vi "Open Log File Instance.vi"(8 "error in (no error)":errorcluster, 11 "Segmented Log in":refnum<class "Segmented Log.lvclass">) -> (0 "error out":errorcluster, 3 "Segmented Log out":refnum<class "Segmented Log.lvclass">)   [LabVIEW 2015, in "Waveform Data Logger Engine.lvlib" / "Segmented Log.lvclass"]
doc: "This VI opens a new log file instance based on the Log File Specification if the max number of instances has not yet been reached. This VI also notifies any listeners that a new file has been opened. If the max number of instances has already been met, this VI throws an error.\n\nBefore opening the file this VI updates the Instance and CrashFileInstance path tags. The Instance tag represents the one-based file index that the segmented log is about to open. The CrashFileInstance is a number that toggles between one and two. Using this tag allows users to create a crash log file session, which always records a running set of the most recent data to file, so that the last N samples are available in the case of a crash."
uses:
  Segmented Log.lvclass
  Shared/Classes/Log File Specifications/Log File Specification/Log File Specification.lvclass
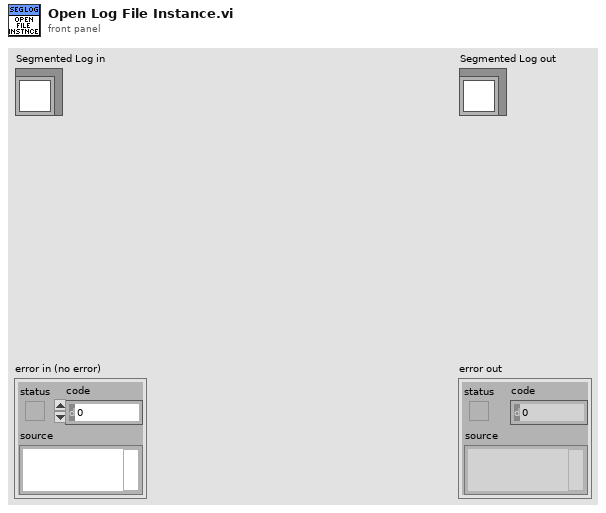
[diagram p1: front panel]
types:
  T1 = typedef "Waveform Data Logger Engine.lvlib/Segmented Log.lvclass/File Open Event Registration.ctl" = cluster{"Callback":refnum<vi>, "User Data":variant}
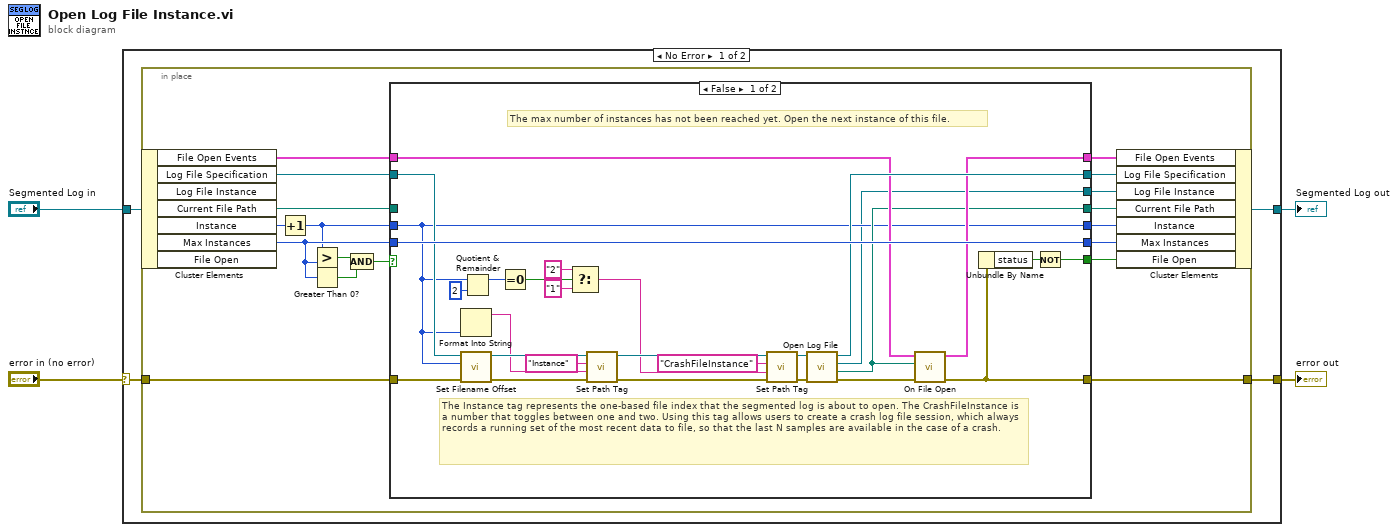
[diagram p0: block diagram]
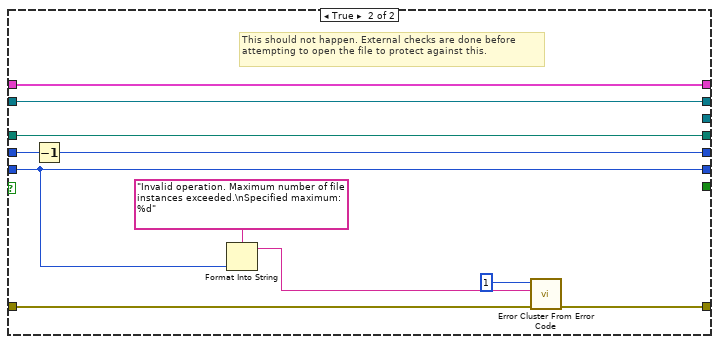
[diagram p2: hidden frame]
diagram:
  n1 = case shown="No Error" "error in (no error)" {
    selector: "error in (no error)" -> [w8 w67]
    tunnel: [w7 w67] -> w3
    tunnel: [w5 w66] -> w1
    tunnel: "Segmented Log in" -> [w6 w66]
    frame No Error {
      n2 = in-place {
        in-place-border: w8 -> [w25]
        in-place-border: [w20] -> w7
        n3 = in-place-cluster #1(w6) -> ("File Open Events"=w10:T1[], "Log File Specification"=w19:refnum<class "Log File Specification.lvclass">, "Current File Path"=w18:path, "Instance"=w14:i32, "Max Instances"=w26:i32)  [unwired: 2 out]
        n4 = Increment(x=w14) -> (x+1=w24:i32)
        n5 = Greater?(x=w24, y=w26) -> (0:w23:bool)
        n6 = Greater Than 0?(x=w26) -> (x > 0?=w22:bool)
        n7 = Compound Arithmetic op=AND(w23, w22) -> (w21:bool)
        n8 = case shown="False" w21 {
          tunnel: w25 -> [w44 w65]
          tunnel: w24 -> [w34 w57]
          tunnel: [w53 w61] -> w20
          tunnel: w26 -> [w52 w60]
          tunnel: w19 -> [w41 w59]
          tunnel: w18 -> [_ w58]
          tunnel: [w46 w58] -> w17
          tunnel: [w49 w59] -> w16
          tunnel: [w34 w56] -> w15
          tunnel: [w52 w60] -> w13
          tunnel: [w50 _] -> w12
          tunnel: [w47 w55] -> w11
          tunnel: w10 -> [w48 w55]
          tunnel: [w32 _] -> w9
          frame False {
            # "The Instance tag represents the one-based file index that the segmented log is about to open. The CrashFileInstance is a number that toggles between one and two. Using this tag allows users to create a crash log file session, which always records a running set of the most recent data to file, so that the last N samples are available in the case of a crash."
            # "The max number of instances has not been reached yet. Open the next instance of this file."
            n9 = Format Into String(w34) -> (resulting string=w40:string)  [unwired: 3 in, 1 out]
            n10 = call "Set Filename Offset.vi"("error in (no error)"=w44, "Filename Offset"=w34, "Log File Specification in"=w41) -> ("error out"=w43:errorcluster, "Log File Specification out"=w42:refnum<class "Log File Specification.lvclass">)  [unwired: 7 in]
            n11 = Quotient & Remainder(x=w34, y=2) -> (x-y*floor(x/y)=w31:i32)  [unwired: 1 out]
            n12 = Equal To 0?(x=w31) -> (x = 0?=w30:bool)
            n13 = Select(t="2" ("Tag Value"), s=w30, f="1") -> (s? t:f=w27:string)
            n14 = call "Set Path Tag.vi"("error in (no error)"=w43, "Tag Value"=w40, "Tag Name"="Instance", "Log File Specification in"=w42) -> ("error out"=w35:errorcluster, "Log File Specification out"=w36:refnum<class "Log File Specification.lvclass">)  [unwired: 6 in]
            n15 = call "Set Path Tag.vi"("error in (no error)"=w35, "Tag Value"=w27, "Tag Name"="CrashFileInstance", "Log File Specification in"=w36) -> ("error out"=w37:errorcluster, "Log File Specification out"=w38:refnum<class "Log File Specification.lvclass">)  [unwired: 6 in]
            n16 = call "Open Log File.vi"("error in (no error)"=w37, "Log File Specification in"=w38) -> ("error out"=w54:errorcluster, "Instance File Path"=w46:path, "Log File out"=w32:refnum<class "Log File.lvclass">, "Log File Specification out"=w49:refnum<class "Log File Specification.lvclass">)  [unwired: 6 in]
            n17 = call "On File Open.vi"("error in (no error)"=w54, "Path"=w46, "File Open Event Registrations in"=w48) -> ("error out"=w53:errorcluster, "File Open Event Registrations out"=w47:T1[])  [unwired: 7 in]
            n18 = Unbundle By Name(w53) -> ("status"=w51:bool)
            n19 = Not(x=w51) -> (.not. x?=w50:bool)
          }
          frame True {
            # "This should not happen. External checks are done before attempting to open the file to protect against this."
            n20 = Decrement(x=w57) -> (x-1=w56:i32)
            n21 = Format Into String(format string="Invalid operation. Maximum number of file instances exceeded.\nSpecified maximum: %d", w60) -> (resulting string=w62:string)  [unwired: 2 in, 1 out]
            n22 = call <vilib>:"Error Cluster From Error Code.vi"("error in (no error)"=w65, "error message (\"\")"=w62, "error code (0)"=1) -> ("error out"=w61:errorcluster)  [unwired: 6 in]
          }
        }
        n23 = in-place-cluster #1("File Open Events"=w11, "Log File Specification"=w16, "Log File Instance"=w9, "Current File Path"=w17, "Instance"=w15, "Max Instances"=w13, "File Open"=w12) -> (w5:refnum<class "Segmented Log.lvclass">)
      }
    }
    frame Error {
    }
  }
  "error out" <- w3
  "Segmented Log out" <- w1
